vi "InitializeAllDevices.vi"(8 "error in (no error)":errorcluster, 11 "XML File Name":string) -> (0 "error out":errorcluster, 1 "Meter":refnum<class "Meter.lvclass">, 2 "Scope":refnum<class "Scope.lvclass">, 3 "Signal Generator":refnum<class "Signal Generation.lvclass">, 4 "Switch":refnum<class "Switch.lvclass">)   [LabVIEW 2011]
doc: "InitializeAllDevices first configures the switch to test DUT 1 and then reads the xml configuration file to determine the instrument types, hardware resource names, and DSSP class paths. It then dynamically loads the corresponding DSSP classes and calls the Initialize Device instance of each DSSP class. Each Initialize Device opens the hardware resource session and resets the instrument. \nInitializeAllDevices saves the class references in global variables that are used in the other VIs."
uses:
  DSSP Modules/Output Classes/Signal Generation/Signal Generation.lvclass
  DSSP Modules/Input Classes/Scope/Scope.lvclass
  DSSP Modules/Input Classes/Meter/Meter.lvclass
  DSSP Modules/Output Classes/Switch/Switch.lvclass
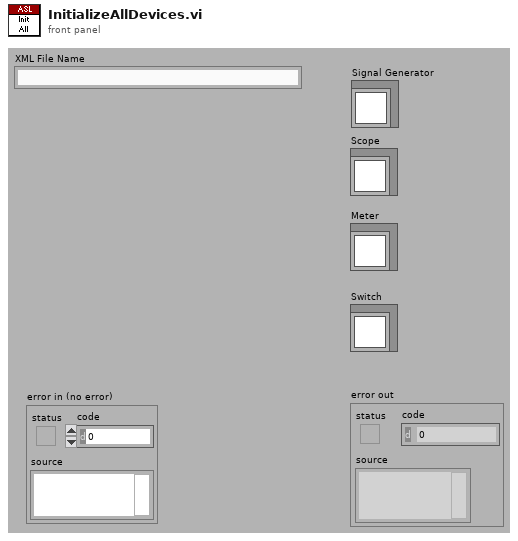
[diagram p1: front panel]
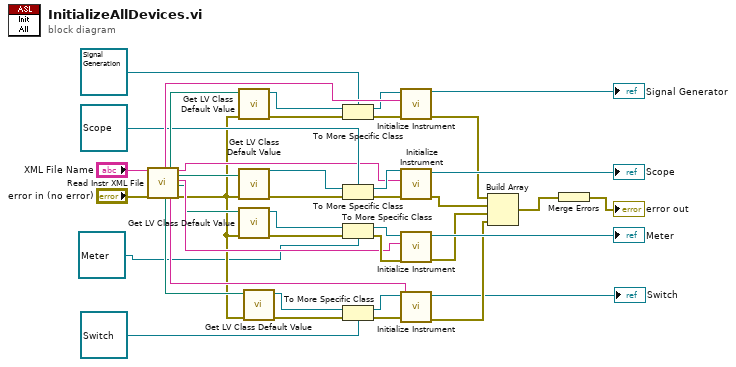
[diagram p0: block diagram]
diagram:
  n1 = call "Read Instr XML File.vi"("XML File Name"="XML File Name", "error in (no error)"="error in (no error)") -> ("Instr 1 Resource Str"=w41:string, "Instr 4 Class Path"=w13:path, "Instr 1 Class Path"=w40:path, "Instr 4 Resource Str"=w14:string, "Instr 2 Resource Str"=w18:string, "Instr 2 Class Path"=w17:path, "Instr 3 Resource Str"=w16:string, "Instr 3 Class Path"=w15:path, "error IO"=w12:errorcluster)  [unwired: 9 out]
  n2 = call <vilib>:"Get LV Class Default Value.vi"("error in (no error)"=w12, "class path"=w40) -> ("error out"=w35:errorcluster, "object"=w39:refnum<class>)  [unwired: 8 out]
  n3 = call <vilib>:"Get LV Class Default Value.vi"("error in (no error)"=w12, "class path"=w17) -> ("error out"=w33:errorcluster, "object"=w38:refnum<class>)  [unwired: 8 out]
  n4 = call <vilib>:"Get LV Class Default Value.vi"("error in (no error)"=w12, "class path"=w15) -> ("error out"=w30:errorcluster, "object"=w31:refnum<class>)  [unwired: 8 out]
  n5 = call <vilib>:"Get LV Class Default Value.vi"("error in (no error)"=w12, "class path"=w13) -> ("error out"=w20:errorcluster, "object"=w19:refnum<class>)  [unwired: 8 out]
  n6 = To More Specific Class(target class=refnum<class "Signal Generation.lvclass"> refnum ("Signal Generation.lvclass"), reference=w39, error in=w35) -> (specific class reference=w37:refnum<class "Signal Generation.lvclass">, error out=w34:errorcluster)
  n7 = To More Specific Class(target class=refnum<class "Scope.lvclass"> refnum ("Scope.lvclass"), reference=w38, error in=w33) -> (specific class reference=w36:refnum<class "Scope.lvclass">, error out=w32:errorcluster)
  n8 = To More Specific Class(target class=refnum<class "Meter.lvclass"> refnum ("Meter.lvclass"), reference=w31, error in=w30) -> (specific class reference=w27:refnum<class "Meter.lvclass">, error out=w28:errorcluster)
  n9 = To More Specific Class(target class=refnum<class "Switch.lvclass"> refnum ("Switch.lvclass"), reference=w19, error in=w20) -> (specific class reference=w3:refnum<class "Switch.lvclass">, error out=w21:errorcluster)
  n10 = call-dynamic "Initialize Instrument.vi"("error in (no error)"=w34, "Instr Resource Str"=w41, "DSSP.lvclass in"=w37) -> ("error out"=w11:errorcluster, "DSSP.lvclass out"=→"Signal Generator":refnum<class "Signal Generation.lvclass">)  [unwired: 7 out]
  n11 = call-dynamic "Initialize Instrument.vi"("error in (no error)"=w32, "Instr Resource Str"=w18, "DSSP.lvclass in"=w36) -> ("error out"=w10:errorcluster, "DSSP.lvclass out"=→"Scope":refnum<class "Scope.lvclass">)  [unwired: 7 out]
  n12 = call-dynamic "Initialize Instrument.vi"("error in (no error)"=w28, "Instr Resource Str"=w16, "DSSP.lvclass in"=w27) -> ("error out"=w9:errorcluster, "DSSP.lvclass out"=→"Meter":refnum<class "Meter.lvclass">)  [unwired: 7 out]
  n13 = call-dynamic "Initialize Instrument.vi"("error in (no error)"=w21, "Instr Resource Str"=w14, "DSSP.lvclass in"=w3) -> ("error out"=w8:errorcluster, "DSSP.lvclass out"=→"Switch":refnum<class "Switch.lvclass">)  [unwired: 7 out]
  n14 = Build Array(w11, w10, w9, w8) -> (w6:errorcluster[])
  n15 = Merge Errors(w6) -> (→"error out":errorcluster)
